vi "niRFUtil FTW Generate Gaussian Response.vi"(2 "Minimum Selectivity (dB)":dbl=70.0 format="%.2f", 3 "df (Hz)":dbl format="%^.2e", 4 "Bandwidth (Hz)":T3 format="%^.3e", 5 "Center Frequency (Hz)":dbl format="%^.6e") -> (0 "-ENBW (dB-Hz)":sgl format="%.2f", 1 "Filter Power Response":T1 {"y" min=0 max=127 format="%.2f"; "dx" format="%^.2e"; "x0" format="%^.2e"})   [LabVIEW 2015, in "niRFUtil.lvlib"]
doc: "(c) Copyright 2006, National Instruments, Inc. This VI may not be duplicated, sold, or distributed without written consent from National Instruments."
uses:
  niRFUtil.lvlib
  Includes/niRFUtil INC RBW Filter Bandwidth.ctl
  Includes/niRFUtil INC Real Waveform.ctl
  Includes/niRFUtil INC Real Array.ctl
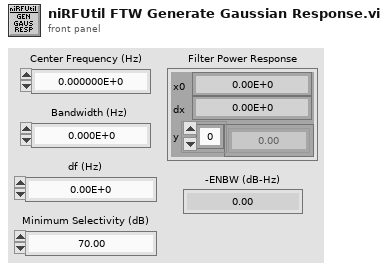
[diagram p1: front panel]
types:
  T1 = typedef "niRFUtil.lvlib/niRFUtil INC Real Waveform.ctl" = cluster{"x0":dbl, "dx":dbl, "y":T2}
  T2 = typedef "niRFUtil.lvlib/niRFUtil INC Real Array.ctl" = sgl[]
  T3 = typedef "niRFUtil.lvlib/niRFUtil INC RBW Filter Bandwidth.ctl" = dbl
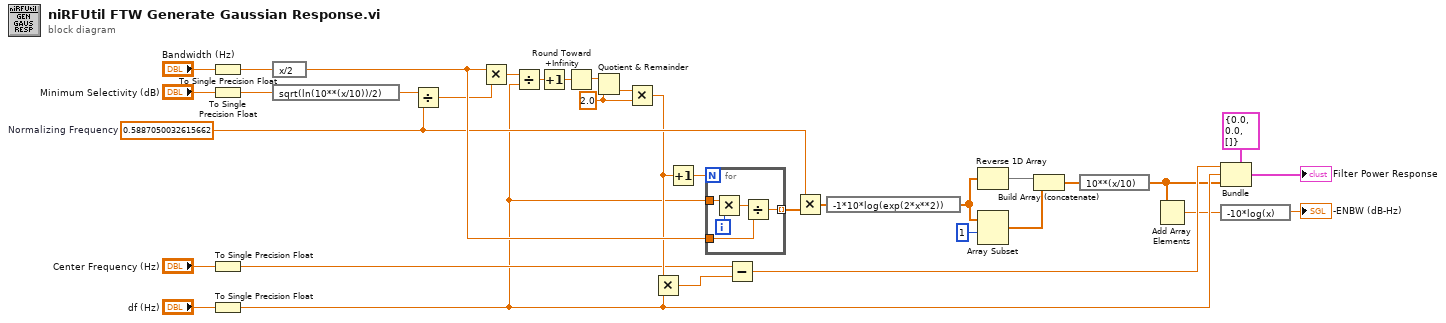
[diagram p0: block diagram]
diagram:
  w16 = sgl 2.0 ("y")
  w20 = sgl 0.588705  # Normalizing Frequency
  n1 = To Single Precision Float(number="Bandwidth (Hz)") -> (single precision float=w5:sgl)
  n2 = To Single Precision Float(number="Minimum Selectivity (dB)") -> (single precision float=w4:sgl)
  n3 = To Single Precision Float(number="Center Frequency (Hz)") -> (single precision float=w7:sgl)
  n4 = To Single Precision Float(number="df (Hz)") -> (single precision float=w6:sgl)
  n5 = expression code="x/2"(w5) -> (w27:sgl)
  n6 = expression code="sqrt(ln(10**(x/10))/2)"(w4) -> (w24:sgl)
  n7 = Divide(x=w24, y=w20) -> (x/y=w23:sgl)
  n8 = Multiply(x=w27, y=w23) -> (x*y=w30:sgl)
  n9 = Divide(x=w30, y=w6) -> (x/y=w19:sgl)
  n10 = Increment(x=w19) -> (x+1=w14:sgl)
  n11 = Round Toward +Infinity(x=w14) -> (ceil(x): smallest int >= x=w18:sgl)
  n12 = Quotient & Remainder(x=w18, y=w16) -> (floor(x/y)=w17:sgl)  [unwired: 1 out]
  n13 = Multiply(x=w17, y=w16) -> (x*y=w15:sgl)
  n14 = Multiply(x=w15, y=w6) -> (x*y=w26:sgl)
  n15 = Increment(x=w15) -> (x+1=w28:sgl)
  n16 = for {
    N: w28 -> [_]
    tunnel: w6 -> [w39]
    tunnel: w27 -> [w36]
    tunnel: [w35] -> w21 mode=indexing
    i -> [w38]
    n17 = Multiply(x=w39, y=w38) -> (x*y=w37:sgl)
    n18 = Divide(x=w37, y=w36) -> (x/y=w35:sgl)
  }
  n19 = Subtract(x=w7, y=w26) -> (x-y=w10:sgl)
  n20 = Multiply(x=w20, y=w21) -> (x*y=w22:sgl[])
  n21 = expression code="-1*10*log(exp(2*x**2))"(w22) -> (w25:sgl[])
  n22 = Reverse 1D Array(array=w25) -> (reversed array=w13:sgl[])
  n23 = Array Subset(array=w25, index=1) -> (w12:sgl[])  [unwired: 1 in]
  n24 = Build Array (concatenate)(w13, w12) -> (w11:sgl[])
  n25 = expression code="10**(x/10)"(w11) -> (w2:sgl[])
  n26 = Add Array Elements(numeric array=w2) -> (sum=w3:sgl)
  n27 = Bundle(cluster=T1 {"x0"=0.0, "dx"=0.0, "y"=[]} ("Filter"), "x0"=w10, "dx"=w6, "y"=w2) -> (→"Filter Power Response":T1)
  n28 = expression code="-10*log(x)"(w3) -> (→"-ENBW (dB-Hz)":sgl)
